vi "PROJECT_LABVIEW.vi"() -> ()   [LabVIEW 2020]
uses:
  <vilib>/Utility/NIReport.llb/Report Type.ctl
  <vilib>/DAQmx/write.llb/DAQmx Write (Analog Wfm 1Chan NSamp).vi
  <vilib>/DAQmx/read.llb/DAQmx Read (Analog 1D Wfm NChan NSamp).vi
  <vilib>/DAQmx/create/channels.llb/DAQmx Create Channel (AO-Voltage-Basic).vi
  <vilib>/DAQmx/configure/timing.llb/DAQmx Timing (Sample Clock).vi
  <vilib>/DAQmx/create/channels.llb/DAQmx Create Channel (AI-Voltage-Basic).vi
  <vilib>/DAQmx/miscellaneous.llb/DAQmx Fill In Error Info.vi
  <vilib>/measure/mascope.llb/Amplitude and Levels 1 chan.vi
  <vilib>/measure/madcrms.llb/Basic Averaged DC-RMS for 1 Chan.vi
  <vilib>/Utility/NIReport.llb/Append Report Text (str wrap).vi
  <vilib>/measure/maspectr.llb/FFT Spectrum (Mag-Phase) for 1 Chan.vi
  <vilib>/Utility/NIReport.llb/NI_report.lvclass
  <vilib>/measure/NI_MABase.lvlib
  <vilib>/measure/NI_MAPro.lvlib
  <resource>/objmgr/daqmx.rc
  <vilib>/Utility/NIReport.llb/NI_ReportGenerationCore.lvlib
panel:
  in  "error in 9":errorcluster caption="error in"
  in  "error in 8":errorcluster caption="error in"
  in  "error in 7":errorcluster caption="error in"
  in  "Tab Control":T1(tab)
  in  "number of samples 6":i32=1000
  in  "rate 6":dbl=1000.0 format="%0.2f"
  out "Generated signal (input) 6":waveform(dbl)(graph)
  in  "amplitude 6":dbl=1.0 format="%0.2p"
  in  "frequency 6":dbl=10.0 format="%0.2p"
  out "VL ARRAY 6":dbl[](array[numeric])
  in  "ADD MEASURMENT 6":bool
  out "IL 6":dbl[](array[numeric])
  in  "Current RL":dbl
  out "VS 6":dbl[](graph)
  out "VL 6":dbl[](graph)
  in  "stop 6":bool
  in  "(6) student ID 2":string
  in  "(6) student name  2":string
  in  "(6) additional comment":string
  out "Date and time 11":string
  in  "(6) student name  1":string
  in  "(6) student ID  1":string
  out "Date and time 10":string
  in  "(5) additional comment":string
  in  "(5) student ID  1":string
  in  "(5) student name  1":string
  in  "(5) student name  2":string
  in  "(5) student ID 2":string
  out "VL 5 VS IL 5":cluster{dbl[], dbl[]}(graph)
  in  "number of samples 5":i32=1000
  in  "rate 5":dbl=1000.0 format="%0.2f"
  in  "amplitude 5":dbl=1.0 format="%0.2p"
  in  "frequency 5":dbl=10.0 format="%0.2p"
  in  "ADD MEASURMENT":bool
  out "IL 5":dbl[](array[numeric])
  in  "Current RL":dbl
  out "VL 5":dbl[](array[numeric])
  out "VS-VL":dbl[](array[numeric])
  in  "CREATE REPORT 5":bool
  out "VL 5":waveform(dbl)(graph)
  out "Output (time) 3":waveform(dbl)(graph)
  out "Input(time) 3":waveform(dbl)(graph)
  out "Common gain 3":dbl[](graph)
  in  "number of samples 3":i32=1000
  in  "rate 6":dbl=1000.0
  out "frequency of sine 3":i32
  in  "amplitude 6":dbl=1.0 format="%0.2p"
  in  "From[hz] 3":i32
  in  "No of points 3":i32
  in  "To[hz] 3":i32
  in  "(3) student ID 2":string
  in  "(3) student name  2":string
  in  "(3) student name  1":string
  in  "(3) student ID  1":string
  in  "(3) additional comment  2":string
  out "Date and time 9":string
  in  "number of samples 2":i32=1000
  in  "rate 2":dbl=1000.0
  out "frequency of sine 2":i32
  in  "From[hz] 2":i32
  in  "No of points 2":i32
  in  "amplitude 2":dbl=1.0 format="%0.2p"
  in  "To[hz] 2":i32
  out "Diffrential gain 2":dbl[](graph)
  out "Output (time) 2":waveform(dbl)(graph)
  out "Input(time) 2":waveform(dbl)(graph)
  in  "(2) student ID 2":string
  in  "(2) student name 2":string
  in  "(2) student name  1":string
  in  "(2) student ID 1":string
  in  "(2) additional comment":string
  out "Date and time 8":string
  # "Report generator"
  # "Max current"
  # "Function generator"
  # "Report generator"
  # "Function generator"
  # "Output Resistance"
  # "Common mode gain"
  # "Connect output zero to Output \nConnect output to Input"
  # "Function generator"
  # "The generated signal in sweep is output1"
  # "Frequency sweep"
  # "Report generator"
  # "Differential amplification and bandwidth measurment"
  # "Connect output zero to Output \nConnect output one to Input\nThe generated signal in sweep is output1"
  # "Function generator"
  # "Frequency sweep"
  # "Report generator"
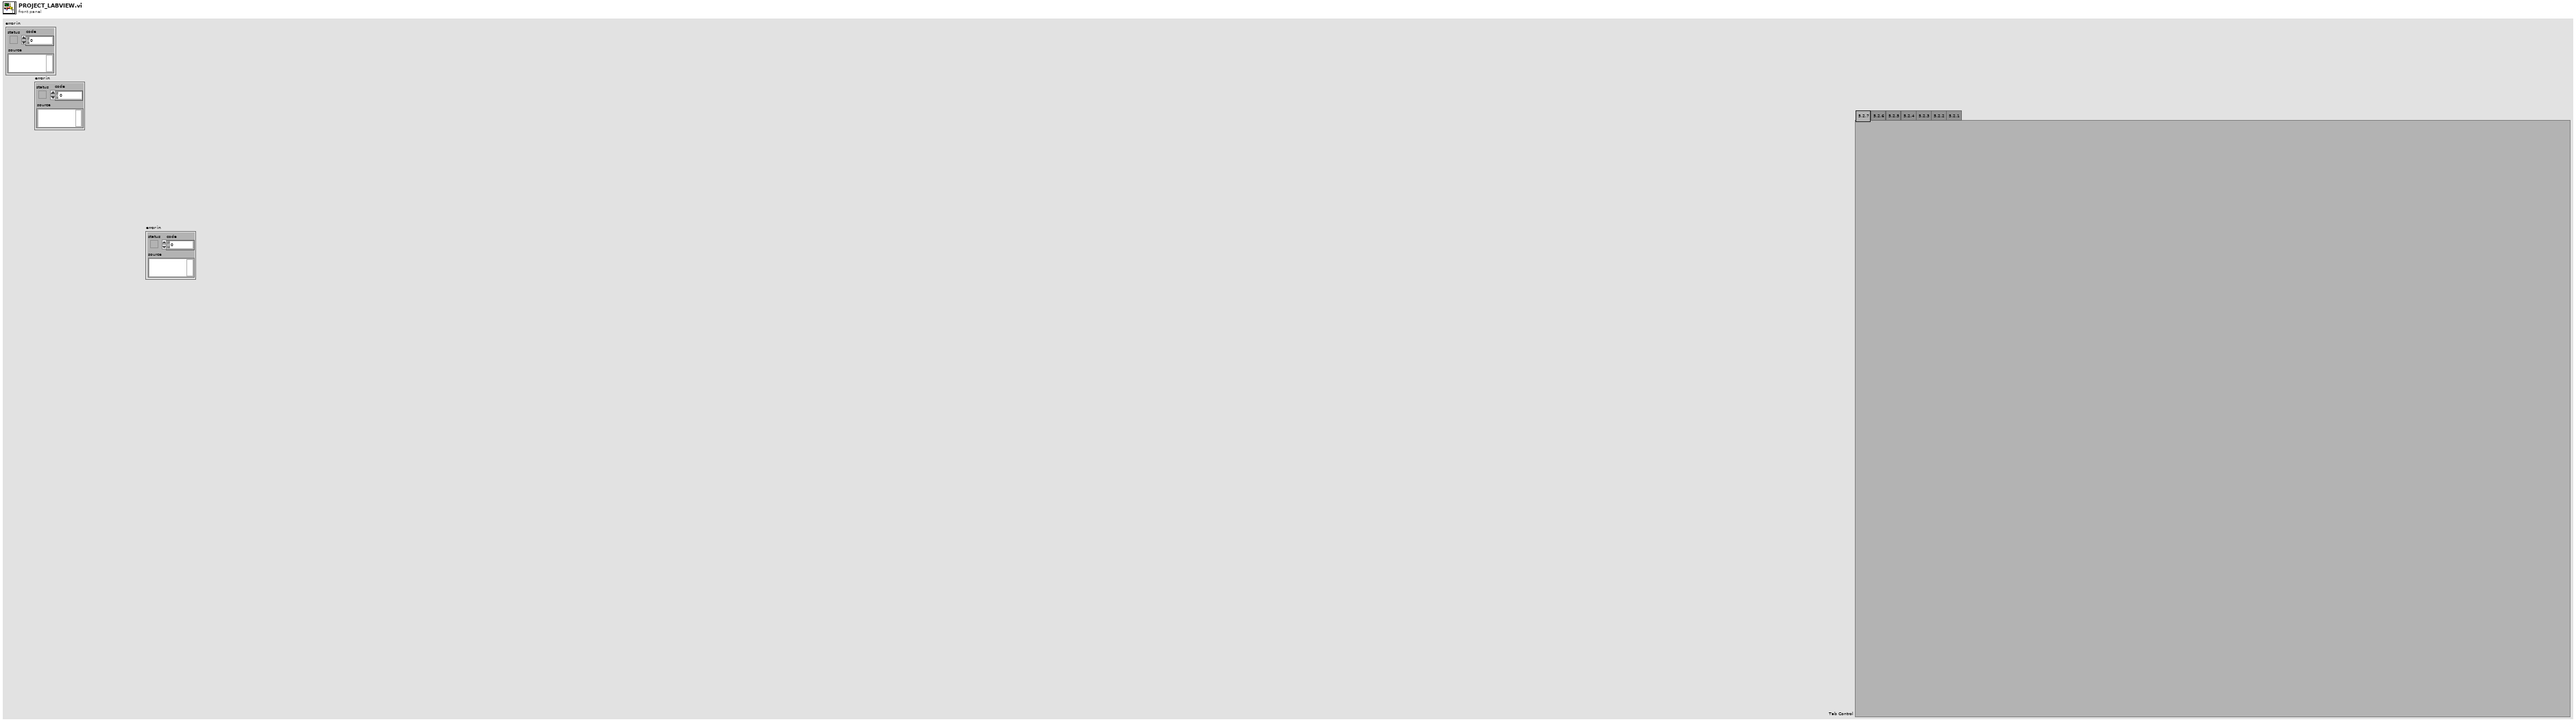
[diagram p1: front panel]
types:
  T1 = enum32{"5.2.7", "5.2.6", "5.2.5", "5.2.4", "5.2.3", "5.2.2", "5.2.1"}
  T2 = typedef "NI_ReportGenerationCore.lvlib/Report Type.ctl" = enum16{"HTML", "Word", "Excel"}
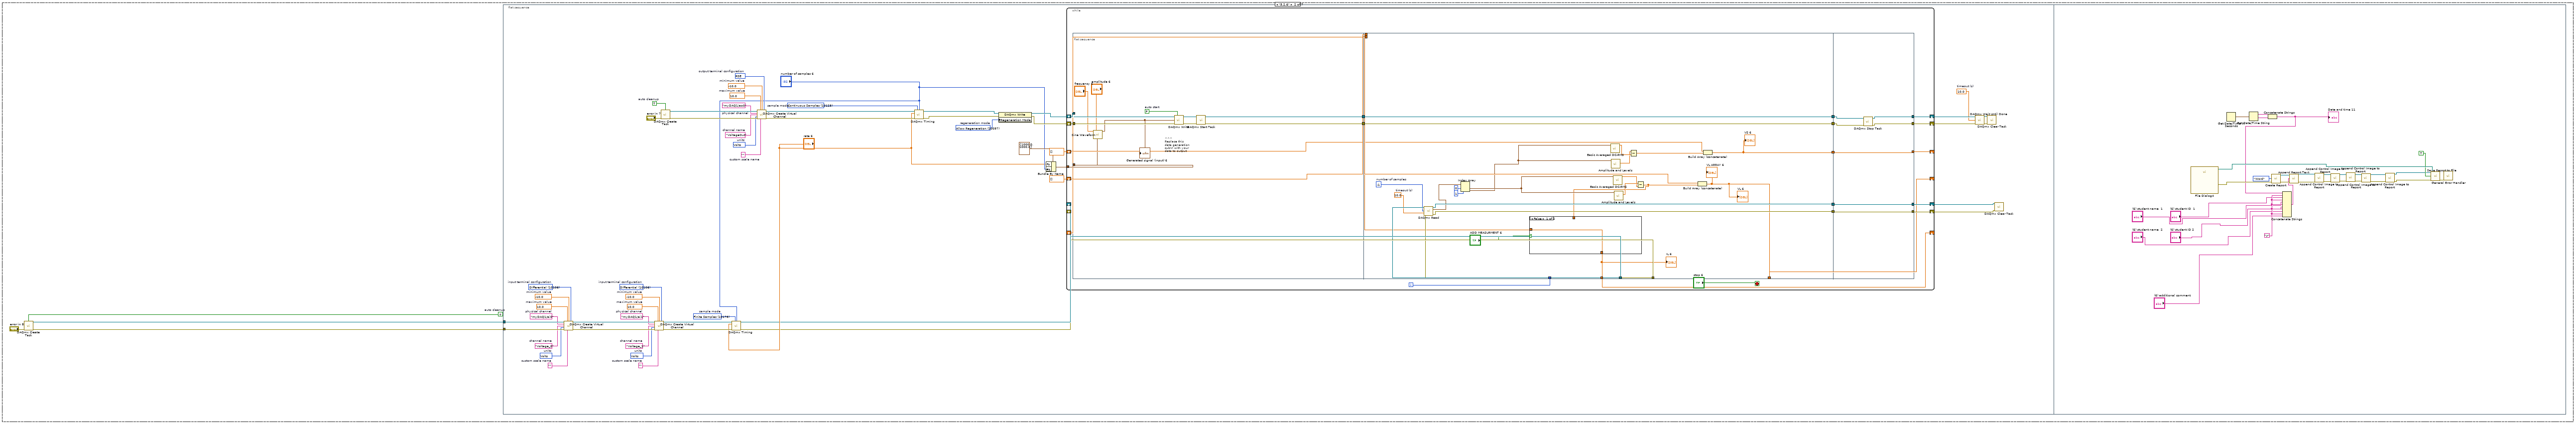
[diagram p3: hidden frame]
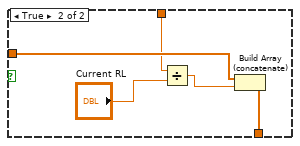
[diagram p4: hidden frame]
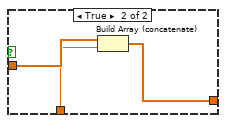
[diagram p6: hidden frame]
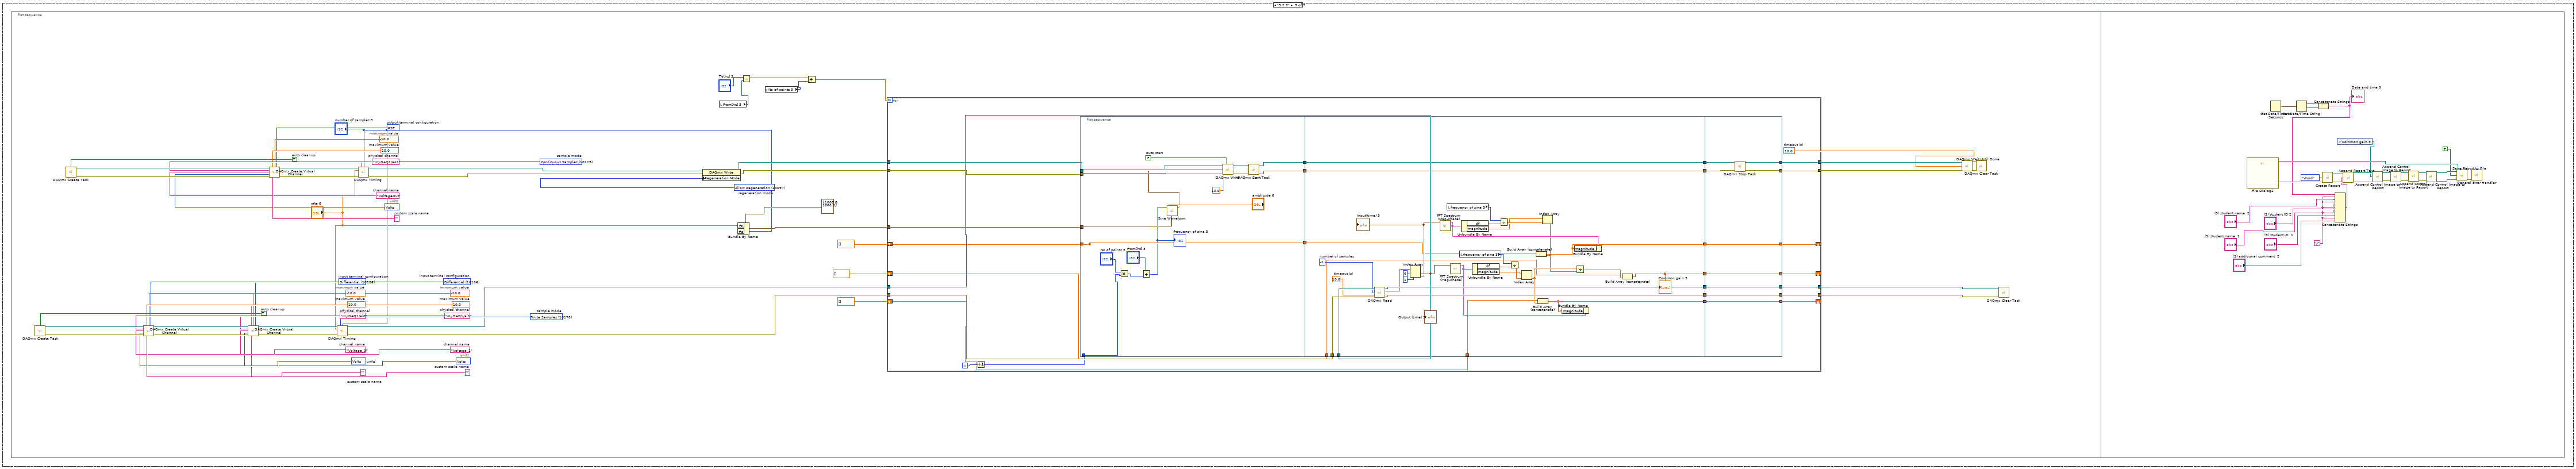
[diagram p9: hidden frame]
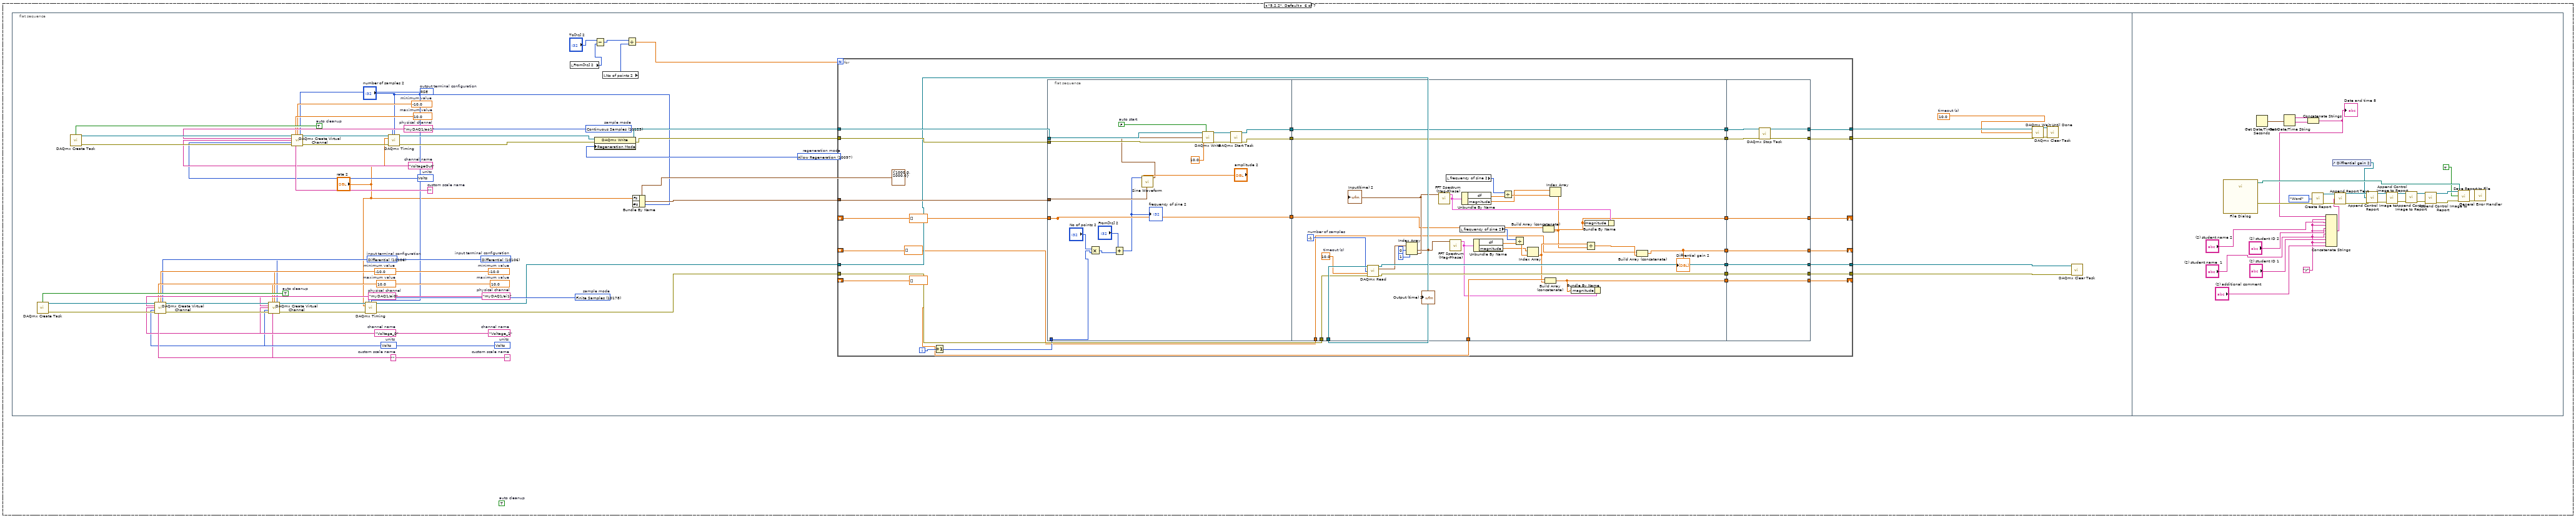
[diagram p10: hidden frame]
diagram:
  n1 = case shown="\"5.2.5\"" "Tab Control" {
    frame "5.2.7" {
    }
    frame "5.2.6" {
      w3 = TRUE  # auto cleanup
      n2 = call <vilib>:"DAQmx Create Task.vi"("auto cleanup"=w3, "error in"="error in 8") -> ("task out"=w2:refnum<k21>, "error out"=w4:errorcluster)  [unwired: 12 in]
      n3 = flat-sequence {
        tunnel: w4 -> [w35]
        tunnel: w2 -> [w34]
        frame #0 {
          w6 = 10.0  # timeout (s)
          w15 = 10178 items=["Finite Samples"=10178, "Continuous Samples"=10123, "Hardware Timed Single Point"=12522]  # sample mode
          w17 = 10106 items=["default"=-1, "RSE"=10083, "NRSE"=10078, "Differential"=10106, "Pseudodifferential"=12529]  # input terminal configuration
          w18 = 10348 items=["Volts"=10348, "From Custom Scale"=10065]  # units
          w19 = "Voltage_1"  # channel name
          w21 = ""  # custom scale name
          w22 = -10.0  # minimum value
          w23 = 10.0  # maximum value
          w24 = "myDAQ1/ai1"  # physical channel
          w26 = 10106 items=["default"=-1, "RSE"=10083, "NRSE"=10078, "Differential"=10106, "Pseudodifferential"=12529]  # input terminal configuration
          w27 = 10348 items=["Volts"=10348, "From Custom Scale"=10065]  # units
          w28 = "Voltage_0"  # channel name
          w30 = ""  # custom scale name
          w31 = -10.0  # minimum value
          w32 = 10.0  # maximum value
          w33 = "myDAQ1/ai0"  # physical channel
          w44 = 10097 items=["Allow Regeneration"=10097, "Do Not Allow Regeneration"=10158]  # regeneration mode
          w46 = 10123 items=["Finite Samples"=10178, "Continuous Samples"=10123, "Hardware Timed Single Point"=12522]  # sample mode
          w49 = 10083 items=["Default"=-1, "RSE"=10083, "Differential"=10106, "Pseudodifferential"=12529]  # output terminal configuration
          w50 = 10348 items=["Volts"=10348, "From Custom Scale"=10065]  # units
          w51 = "VoltageOut"  # channel name
          w53 = ""  # custom scale name
          w54 = -10.0  # minimum value
          w55 = 10.0  # maximum value
          w56 = "myDAQ1/ao0"  # physical channel
          w58 = TRUE  # auto cleanup
          n4 = call-poly <vilib>:"DAQmx Create Virtual Channel.vi"("task in"=w34, "maximum value"=w32, "minimum value"=w31, "input terminal configuration"=w26, "physical channels"=w33, "name to assign"=w28, "units"=w27, "error in"=w35, "custom scale name"=w30) -> ("task out"=w25:refnum<k21>, "error out"=w29:errorcluster)  [unwired: 5 in]
          n5 = call-poly <vilib>:"DAQmx Create Virtual Channel.vi"("task in"=w25, "maximum value"=w23, "minimum value"=w22, "input terminal configuration"=w17, "physical channels"=w24, "name to assign"=w19, "units"=w18, "error in"=w29, "custom scale name"=w21) -> ("task out"=w16:refnum<k21>, "error out"=w20:errorcluster)  [unwired: 5 in]
          n6 = call <vilib>:"DAQmx Create Task.vi"("auto cleanup"=w58, "error in"="error in 7") -> ("task out"=w57:refnum<k21>, "error out"=w59:errorcluster)  [unwired: 12 in]
          n7 = call-poly <vilib>:"DAQmx Timing.vi"("task/channels in"=w16, "sample mode"=w15, "samples per channel"="number of samples 6", "rate"="rate 6", "error in"=w20) -> ("task out"=w12:refnum<k21>, "error out"=w11:errorcluster)  [unwired: 9 in]
          n8 = call-poly <vilib>:"DAQmx Create Virtual Channel.vi"("task in"=w57, "maximum value"=w55, "minimum value"=w54, "output terminal configuration"=w49, "physical channels"=w56, "name to assign"=w51, "units"=w50, "error in"=w59, "custom scale name"=w53) -> ("task out"=w47:refnum<k21>, "error out"=w52:errorcluster)  [unwired: 5 in]
          n9 = call-poly <vilib>:"DAQmx Timing.vi"("task/channels in"=w47, "sample mode"=w46, "samples per channel"="number of samples 6", "rate"="rate 6", "error in"=w52) -> ("task out"=w45:refnum<k21>, "error out"=w48:errorcluster)  [unwired: 9 in]
          n10 = property class="DAQmx Write"(reference=w45, error in=w48, "Regeneration Mode"=w44) -> (reference out=w43:refnum<k21>, error out=w42:errorcluster)
          n11 = Bundle By Name(cluster=cluster{"Fs":dbl, "#s":dbl} {"Fs"=1000.0, "#s"=1000.0} ("sampling info"), "Fs"="rate 6", "#s"="number of samples 6") -> (w36:cluster{"Fs":dbl, "#s":dbl})
          n12 = while {
            tunnel: w36 -> [w74]
            shift-right: [w76] -> w39
            shift-left: w43 -> [w78]
            shift-right: [w75] -> w38
            shift-left: w42 -> [w77]
            shift-right: [w71] -> w10
            shift-left: w12 -> [w73]
            shift-right: [w70] -> w9
            shift-left: w11 -> [w72]
            shift-right: [w68] -> _
            shift-left: dbl[] [] -> [w65]
            shift-right: [w67] -> _
            shift-left: dbl[] [] -> [w66]
            shift-right: [w63] -> _
            shift-left: _ -> [w62]
            i -> [w64]
            stop <- "stop 6" stop-if-true
            n13 = flat-sequence {
              tunnel: w78 -> [w92]
              tunnel: w77 -> [w91]
              tunnel: [w90] -> w84
              tunnel: [w89] -> w83
              tunnel: w74 -> [w86]
              tunnel: w84 -> [w121]
              tunnel: [w121] -> w82
              tunnel: w83 -> [w120]
              tunnel: [w120] -> w81
              tunnel: w73 -> [w119]
              tunnel: w72 -> [w118]
              tunnel: [w115] -> w80
              tunnel: [w114] -> w79
              tunnel: [w103] -> w69
              tunnel: [w102] -> w67
              tunnel: w66 -> [w105]
              tunnel: w65 -> [w104]
              tunnel: w64 -> [_]
              tunnel: [w99] -> w63
              tunnel: w62 -> [w98]
              tunnel: [w131] -> w75
              tunnel: [w132] -> w76
              tunnel: w82 -> [w134]
              tunnel: w81 -> [w133]
              tunnel: w80 -> [w130]
              tunnel: w79 -> [w129]
              tunnel: [w130] -> w71
              tunnel: [w129] -> w70
              tunnel: w69 -> [w128]
              tunnel: [w128] -> w68
              frame #0 {
                w95 = FALSE  # auto start
                # "^^^\nReplace this\ndata generation\nsubVI with your\ndata to output"
                n14 = call <vilib>:"Sine Waveform.vi"("sampling info"=w86, "amplitude"="amplitude 6", "frequency"="frequency 6") -> ("signal out"=w85:waveform(dbl))  [unwired: 7 in, 1 out]
                "Generated signal (input) 6" <- w85
                n15 = call-poly <vilib>:"DAQmx Write.vi"("task/channels in"=w92, "auto start"=w95, "data"=w85, "error in"=w91) -> ("task out"=w94:refnum<k21>, "error out"=w93:errorcluster)  [unwired: 9 in, 1 out]
                n16 = call <vilib>:"DAQmx Start Task.vi"("task/channels in"=w94, "error in"=w93) -> ("task out"=w90:refnum<k21>, "error out"=w89:errorcluster)  [unwired: 12 in]
              }
              frame #1 {
                w116 = 10.0  # timeout (s)
                w117 = -1  # number of samples
                n17 = call-poly <vilib>:"DAQmx Read.vi"("task/channels in"=w119, "number of samples per channel"=w117, "timeout"=w116, "error in"=w118) -> ("task out"=w115:refnum<k21>, "data"=w113:waveform(dbl)[], "error out"=w114:errorcluster)  [unwired: 9 in]
                n18 = Index Array(array=w113, index #1=0 ("index"), index #2=1 ("index")) -> (element #1=w101:waveform(dbl), element #2=w100:waveform(dbl))
                n19 = call-poly <vilib>:"Basic Averaged DC-RMS.vi"("signal in"=w100) -> ("DC value"=w108:dbl)  [unwired: 7 in, 3 out]
                n20 = call-poly <vilib>:"Amplitude and Levels.vi"("signal in"=w100) -> ("high state level"=w107:dbl)  [unwired: 7 in, 3 out]
                n21 = call-poly <vilib>:"Basic Averaged DC-RMS.vi"("signal in"=w101) -> ("DC value"=w109:dbl)  [unwired: 7 in, 3 out]
                n22 = call-poly <vilib>:"Amplitude and Levels.vi"("signal in"=w101) -> ("high state level"=w110:dbl)  [unwired: 7 in, 3 out]
                n23 = Subtract(x=w107, y=w108) -> (x-y=w106:dbl)
                n24 = Subtract(x=w110, y=w109) -> (x-y=w96:dbl)
                n25 = case shown="False" "ADD MEASURMENT 6" {
                  tunnel: [w122 w127] -> w99
                  tunnel: w98 -> [w122 w126]
                  tunnel: w96 -> [_ w125]
                  frame False {
                  }
                  frame True {
                    n26 = Divide(x=w125, y="Current RL") -> (x/y=w124:dbl)
                    n27 = Build Array (concatenate)(w126, w124) -> (w127:dbl[])
                  }
                }
                "IL 6" <- w99
                n28 = Build Array (concatenate)(w105, w96) -> (w102:dbl[])
                "VL 6" <- w102
                "VL ARRAY 6" <- w102
                n29 = Build Array (concatenate)(w104, w106) -> (w103:dbl[])
                "VS 6" <- w103
              }
              frame #2 {
                n30 = call <vilib>:"DAQmx Stop Task.vi"("task/channels in"=w134, "error in"=w133) -> ("task out"=w132:refnum<k21>, "error out"=w131:errorcluster)  [unwired: 12 in]
              }
            }
          }
          n31 = call <vilib>:"DAQmx Wait Until Done.vi"("task/channels in"=w39, "timeout (sec)"=w6, "error in"=w38) -> ("task out"=w41:refnum<k21>, "error out"=w40:errorcluster)  [unwired: 11 in]
          n32 = call <vilib>:"DAQmx Clear Task.vi"("task in"=w41, "error in"=w40) -> ()  [unwired: 13 in, 1 out]
          n33 = call <vilib>:"DAQmx Clear Task.vi"("task in"=w10, "error in"=w9) -> ()  [unwired: 13 in, 1 out]
        }
        frame #1 {
          w156 = "\r"
          n34 = call "File Dialog4"() -> ("selected path"=w159:path, "error out"=w158:errorcluster)  [unwired: 12 in, 2 out]
          n35 = Get Date/Time In Seconds() -> (seconds since 1Jan1904=w164:timestamp)
          n36 = Get Date/Time String(seconds (now)=w164) -> (date string=w162:string, time string=w163:string)  [unwired: 2 in]
          n37 = Concatenate Strings(w162, w163) -> (w139:string)
          "Date and time 11" <- w139
          n38 = call <vilib>:"Create Report.vi"("report type"=Report_Type."Word", "error in (no error)"=w158) -> ("report out"=w160:refnum<class "NI_report.lvclass">, "error out"=w161:errorcluster)  [unwired: 12 in]
          n39 = Concatenate Strings(w139, w156, "(6) student ID  1", w156, "(6) student name  1", w156, "(6) student ID 2", w156, "(6) student name  2", w156, "(6) additional comment") -> (w153:string)
          n40 = call-poly <vilib>:"Append Report Text.vi"("report in"=w160, "text"=w153, "error in (no error)"=w161) -> ("report out"=w146:refnum<class "NI_report.lvclass">, "error out"=w145:errorcluster)  [unwired: 9 in, 2 out]
          n41 = call-dynamic "Append Control Image to Report.vi"("report in"=w146, "error in (no error)"=w145) -> ("report out"=w148:refnum<class "NI_report.lvclass">, "error out"=w147:errorcluster)  [unwired: 10 in, 2 out]
          n42 = call-dynamic "Append Control Image to Report.vi"("report in"=w148, "error in (no error)"=w147) -> ("report out"=w149:refnum<class "NI_report.lvclass">, "error out"=w150:errorcluster)  [unwired: 10 in, 2 out]
          n43 = call-dynamic "Append Control Image to Report.vi"("report in"=w149, "error in (no error)"=w150) -> ("report out"=w152:refnum<class "NI_report.lvclass">, "error out"=w151:errorcluster)  [unwired: 10 in, 2 out]
          n44 = call-dynamic "Append Control Image to Report.vi"("report in"=w152, "error in (no error)"=w151) -> ("report out"=w138:refnum<class "NI_report.lvclass">, "error out"=w137:errorcluster)  [unwired: 10 in, 2 out]
          n45 = call-dynamic "Append Control Image to Report.vi"("report in"=w138, "error in (no error)"=w137) -> ("report out"=w136:refnum<class "NI_report.lvclass">, "error out"=w135:errorcluster)  [unwired: 10 in, 2 out]
          n46 = call-dynamic "Save Report to File.vi"("report in"=w136, "report file path"=w159, "prompt to replace? (F)"=TRUE, "error in (no error)"=w135) -> ("error out"=w154:errorcluster)  [unwired: 10 in, 1 out]
          n47 = call <vilib>:"General Error Handler.vi"("error in (no error)"=w154) -> ()  [unwired: 10 in, 5 out]
        }
      }
    }
    frame "5.2.5" {
      w166 = 10106 items=["default"=-1, "RSE"=10083, "NRSE"=10078, "Differential"=10106, "Pseudodifferential"=12529]  # input terminal configuration
      w167 = 10348 items=["Volts"=10348, "From Custom Scale"=10065]  # units
      w168 = "Voltage_0"  # channel name
      w170 = ""  # custom scale name
      w171 = -10.0  # minimum value
      w172 = 10.0  # maximum value
      w173 = "myDAQ1/ai0"  # physical channel
      n48 = call-poly <vilib>:"DAQmx Create Virtual Channel.vi"("maximum value"=w172, "minimum value"=w171, "input terminal configuration"=w166, "physical channels"=w173, "name to assign"=w168, "units"=w167, "custom scale name"=w170) -> ("task out"=w165:refnum<k21>, "error out"=w169:errorcluster)  [unwired: 7 in]
      n49 = flat-sequence {
        tunnel: w169 -> [w191]
        tunnel: w165 -> [w190]
        frame #0 {
          w180 = 10178 items=["Finite Samples"=10178, "Continuous Samples"=10123, "Hardware Timed Single Point"=12522]  # sample mode
          w182 = 10106 items=["default"=-1, "RSE"=10083, "NRSE"=10078, "Differential"=10106, "Pseudodifferential"=12529]  # input terminal configuration
          w183 = 10348 items=["Volts"=10348, "From Custom Scale"=10065]  # units
          w184 = "Voltage_1"  # channel name
          w186 = ""  # custom scale name
          w187 = -10.0  # minimum value
          w188 = 10.0  # maximum value
          w189 = "myDAQ1/ai1"  # physical channel
          w201 = 10097 items=["Allow Regeneration"=10097, "Do Not Allow Regeneration"=10158]  # regeneration mode
          w203 = 10123 items=["Finite Samples"=10178, "Continuous Samples"=10123, "Hardware Timed Single Point"=12522]  # sample mode
          w206 = 10083 items=["Default"=-1, "RSE"=10083, "Differential"=10106, "Pseudodifferential"=12529]  # output terminal configuration
          w207 = 10348 items=["Volts"=10348, "From Custom Scale"=10065]  # units
          w208 = "VoltageOut"  # channel name
          w210 = ""  # custom scale name
          w211 = -10.0  # minimum value
          w212 = 10.0  # maximum value
          w213 = "myDAQ1/ao0"  # physical channel
          w215 = TRUE  # auto cleanup
          n50 = call-poly <vilib>:"DAQmx Create Virtual Channel.vi"("task in"=w190, "maximum value"=w188, "minimum value"=w187, "input terminal configuration"=w182, "physical channels"=w189, "name to assign"=w184, "units"=w183, "error in"=w191, "custom scale name"=w186) -> ("task out"=w181:refnum<k21>, "error out"=w185:errorcluster)  [unwired: 5 in]
          n51 = call <vilib>:"DAQmx Create Task.vi"("auto cleanup"=w215, "error in"="error in 9") -> ("task out"=w214:refnum<k21>, "error out"=w216:errorcluster)  [unwired: 12 in]
          n52 = call-poly <vilib>:"DAQmx Timing.vi"("task/channels in"=w181, "sample mode"=w180, "samples per channel"="number of samples 5", "rate"="rate 5", "error in"=w185) -> ("task out"=w177:refnum<k21>, "error out"=w176:errorcluster)  [unwired: 9 in]
          n53 = call-poly <vilib>:"DAQmx Create Virtual Channel.vi"("task in"=w214, "maximum value"=w212, "minimum value"=w211, "output terminal configuration"=w206, "physical channels"=w213, "name to assign"=w208, "units"=w207, "error in"=w216, "custom scale name"=w210) -> ("task out"=w204:refnum<k21>, "error out"=w209:errorcluster)  [unwired: 5 in]
          n54 = call-poly <vilib>:"DAQmx Timing.vi"("task/channels in"=w204, "sample mode"=w203, "samples per channel"="number of samples 5", "rate"="rate 5", "error in"=w209) -> ("task out"=w202:refnum<k21>, "error out"=w205:errorcluster)  [unwired: 9 in]
          n55 = property class="DAQmx Write"(reference=w202, error in=w205, "Regeneration Mode"=w201) -> (reference out=w200:refnum<k21>, error out=w199:errorcluster)
          n56 = Bundle By Name(cluster=cluster{"Fs":dbl, "#s":dbl} {"Fs"=1000.0, "#s"=1000.0} ("sampling info"), "Fs"="rate 5", "#s"="number of samples 5") -> (w192:cluster{"Fs":dbl, "#s":dbl})
          n57 = while {
            tunnel: [w232] -> w194
            tunnel: w192 -> [w231]
            shift-right: [w234] -> w196
            shift-left: w200 -> [w236]
            shift-right: [w233] -> w195
            shift-left: w199 -> [w235]
            shift-right: [w228] -> w175
            shift-left: w177 -> [w230]
            shift-right: [w227] -> w174
            shift-left: w176 -> [w229]
            shift-right: [w225] -> _
            shift-left: _ -> [w222]
            shift-right: [w224] -> _
            shift-left: _ -> [w223]
            shift-right: [w220] -> _
            shift-left: _ -> [w219]
            i -> [w221]
            stop <- "CREATE REPORT 5" stop-if-true
            w232 = 10.0  # timeout (s)
            n58 = flat-sequence {
              tunnel: w236 -> [w250]
              tunnel: w235 -> [w249]
              tunnel: [w248] -> w242
              tunnel: [w247] -> w241
              tunnel: w231 -> [w244]
              tunnel: w242 -> [w277]
              tunnel: [w277] -> w240
              tunnel: w241 -> [w276]
              tunnel: [w276] -> w239
              tunnel: w230 -> [w275]
              tunnel: w229 -> [w274]
              tunnel: [w271] -> w238
              tunnel: [w270] -> w237
              tunnel: [w260] -> w226
              tunnel: [w254] -> w224
              tunnel: w223 -> [w266]
              tunnel: w222 -> [w265]
              tunnel: w221 -> [_]
              tunnel: [w259] -> w220
              tunnel: w219 -> [w262]
              tunnel: [w295] -> w233
              tunnel: [w296] -> w234
              tunnel: w240 -> [w298]
              tunnel: w239 -> [w297]
              tunnel: w238 -> [w294]
              tunnel: w237 -> [w293]
              tunnel: [w294] -> w228
              tunnel: [w293] -> w227
              tunnel: w226 -> [w292]
              tunnel: [w292] -> w225
              frame #0 {
                w253 = FALSE  # auto start
                # "^^^\nReplace this\ndata generation\nsubVI with your\ndata to output"
                n59 = call <vilib>:"Sine Waveform.vi"("sampling info"=w244, "amplitude"="amplitude 5", "frequency"="frequency 5") -> ("signal out"=w243:waveform(dbl))  [unwired: 7 in, 1 out]
                n60 = call-poly <vilib>:"DAQmx Write.vi"("task/channels in"=w250, "auto start"=w253, "data"=w243, "error in"=w249) -> ("task out"=w252:refnum<k21>, "error out"=w251:errorcluster)  [unwired: 9 in, 1 out]
                n61 = call <vilib>:"DAQmx Start Task.vi"("task/channels in"=w252, "error in"=w251) -> ("task out"=w248:refnum<k21>, "error out"=w247:errorcluster)  [unwired: 12 in]
              }
              frame #1 {
                w272 = 10.0  # timeout (s)
                w273 = -1  # number of samples
                n62 = call-poly <vilib>:"DAQmx Read.vi"("task/channels in"=w275, "number of samples per channel"=w273, "timeout"=w272, "error in"=w274) -> ("task out"=w271:refnum<k21>, "data"=w269:waveform(dbl)[], "error out"=w270:errorcluster)  [unwired: 9 in]
                n63 = Index Array(array=w269, index #1=0 ("index"), index #2=1 ("index")) -> (element #1=w264:waveform(dbl), element #2=w263:waveform(dbl))
                "VL 5" <- w264
                n64 = call-poly <vilib>:"Amplitude and Levels.vi"("signal in"=w264) -> ("amplitude"=w256:dbl)  [unwired: 7 in, 3 out]
                n65 = case shown="True" "ADD MEASURMENT" {
                  tunnel: [w286 w291] -> w259
                  tunnel: w262 -> [w286 w290]
                  tunnel: w256 -> [_ w289]
                  frame False {
                  }
                  frame True {
                    n66 = Divide(x=w289, y="Current RL") -> (x/y=w288:dbl)
                    n67 = Build Array (concatenate)(w290, w288) -> (w291:dbl[])
                  }
                }
                "IL 5" <- w259
                n68 = call-poly <vilib>:"Amplitude and Levels.vi"("signal in"=w263) -> ("amplitude"=w255:dbl)  [unwired: 7 in, 3 out]
                n69 = Subtract(x=w255, y=w256) -> (x-y=w261:dbl)
                n70 = case shown="False" "ADD MEASURMENT" {
                  tunnel: w265 -> [w282 w285]
                  tunnel: w261 -> [_ w284]
                  tunnel: [w282 w283] -> w260
                  frame False {
                  }
                  frame True {
                    n71 = Build Array (concatenate)(w285, w284) -> (w283:dbl[])
                  }
                }
                "VS-VL" <- w260
                n72 = case shown="True" "ADD MEASURMENT" {
                  tunnel: w266 -> [w278 w281]
                  tunnel: [w278 w280] -> w254
                  tunnel: w256 -> [_ w279]
                  frame False {
                  }
                  frame True {
                    n73 = Build Array (concatenate)(w281, w279) -> (w280:dbl[])
                  }
                }
                "VL 5" <- w254
                n74 = Bundle(w254, w259) -> (→"VL 5 VS IL 5":cluster{dbl[], dbl[]})  [unwired: 1 in]
              }
              frame #2 {
                n75 = call <vilib>:"DAQmx Stop Task.vi"("task/channels in"=w298, "error in"=w297) -> ("task out"=w296:refnum<k21>, "error out"=w295:errorcluster)  [unwired: 12 in]
              }
            }
          }
          n76 = call <vilib>:"DAQmx Wait Until Done.vi"("task/channels in"=w196, "timeout (sec)"=w194, "error in"=w195) -> ("task out"=w198:refnum<k21>, "error out"=w197:errorcluster)  [unwired: 11 in]
          n77 = call <vilib>:"DAQmx Clear Task.vi"("task in"=w198, "error in"=w197) -> ()  [unwired: 13 in, 1 out]
          n78 = call <vilib>:"DAQmx Clear Task.vi"("task in"=w175, "error in"=w174) -> ()  [unwired: 13 in, 1 out]
        }
        frame #1 {
          w325 = "\r"
          n79 = call "File Dialog3"() -> ("selected path"=w328:path, "error out"=w327:errorcluster)  [unwired: 12 in, 2 out]
          n80 = Get Date/Time In Seconds() -> (seconds since 1Jan1904=w333:timestamp)
          n81 = Get Date/Time String(seconds (now)=w333) -> (date string=w331:string, time string=w332:string)  [unwired: 2 in]
          n82 = Concatenate Strings(w331, w332) -> (w308:string)
          "Date and time 10" <- w308
          n83 = call <vilib>:"Create Report.vi"("report type"=Report_Type."Word", "error in (no error)"=w327) -> ("report out"=w329:refnum<class "NI_report.lvclass">, "error out"=w330:errorcluster)  [unwired: 12 in]
          n84 = Concatenate Strings(w308, w325, "(5) student ID  1", w325, "(5) student name  1", w325, "(5) student ID 2", w325, "(5) student name  2", w325, "(5) additional comment") -> (w322:string)
          n85 = call-poly <vilib>:"Append Report Text.vi"("report in"=w329, "text"=w322, "error in (no error)"=w330) -> ("report out"=w315:refnum<class "NI_report.lvclass">, "error out"=w314:errorcluster)  [unwired: 9 in, 2 out]
          n86 = control-ref of="IL 5"() -> (w304:refnum<vi>)
          n87 = call-dynamic "Append Control Image to Report.vi"("report in"=w315, "ctrl reference"=w304, "error in (no error)"=w314) -> ("report out"=w317:refnum<class "NI_report.lvclass">, "error out"=w316:errorcluster)  [unwired: 9 in, 2 out]
          n88 = control-ref of="VL 5"() -> (w305:refnum<vi>)
          n89 = call-dynamic "Append Control Image to Report.vi"("report in"=w317, "ctrl reference"=w305, "error in (no error)"=w316) -> ("report out"=w318:refnum<class "NI_report.lvclass">, "error out"=w319:errorcluster)  [unwired: 9 in, 2 out]
          n90 = control-ref of="VS-VL"() -> (w306:refnum<vi>)
          n91 = call-dynamic "Append Control Image to Report.vi"("report in"=w318, "ctrl reference"=w306, "error in (no error)"=w319) -> ("report out"=w321:refnum<class "NI_report.lvclass">, "error out"=w320:errorcluster)  [unwired: 9 in, 2 out]
          n92 = control-ref of="Current RL"() -> (w307:refnum<vi>)
          n93 = call-dynamic "Append Control Image to Report.vi"("report in"=w321, "ctrl reference"=w307, "error in (no error)"=w320) -> ("report out"=w303:refnum<class "NI_report.lvclass">, "error out"=w302:errorcluster)  [unwired: 9 in, 2 out]
          n94 = control-ref of="VL 5 VS IL 5"() -> (w299:refnum<vi>)
          n95 = call-dynamic "Append Control Image to Report.vi"("report in"=w303, "ctrl reference"=w299, "error in (no error)"=w302) -> ("report out"=w301:refnum<class "NI_report.lvclass">, "error out"=w300:errorcluster)  [unwired: 9 in, 2 out]
          n96 = call-dynamic "Save Report to File.vi"("report in"=w301, "report file path"=w328, "prompt to replace? (F)"=TRUE, "error in (no error)"=w300) -> ("error out"=w323:errorcluster)  [unwired: 10 in, 1 out]
          n97 = call <vilib>:"General Error Handler.vi"("error in (no error)"=w323) -> ()  [unwired: 10 in, 5 out]
        }
      }
    }
    frame "5.2.4" {
    }
    frame "5.2.3" {
      n98 = flat-sequence {
        frame #0 {
          w342 = 10.0  # timeout (s)
          w349 = 10178 items=["Finite Samples"=10178, "Continuous Samples"=10123, "Hardware Timed Single Point"=12522]  # sample mode
          w351 = 10106 items=["default"=-1, "RSE"=10083, "NRSE"=10078, "Differential"=10106, "Pseudodifferential"=12529]  # input terminal configuration
          w352 = 10348 items=["Volts"=10348, "From Custom Scale"=10065]  # units
          w353 = "Voltage_1"  # channel name
          w355 = ""  # custom scale name
          w356 = -10.0  # minimum value
          w357 = 10.0  # maximum value
          w358 = "myDAQ1/ai1"  # physical channel
          w360 = 10106 items=["default"=-1, "RSE"=10083, "NRSE"=10078, "Differential"=10106, "Pseudodifferential"=12529]  # input terminal configuration
          w361 = 10348 items=["Volts"=10348, "From Custom Scale"=10065]  # units
          w362 = "Voltage_0"  # channel name
          w364 = ""  # custom scale name
          w365 = -10.0  # minimum value
          w366 = 10.0  # maximum value
          w367 = "myDAQ1/ai0"  # physical channel
          w369 = TRUE  # auto cleanup
          w379 = 10097 items=["Allow Regeneration"=10097, "Do Not Allow Regeneration"=10158]  # regeneration mode
          w381 = 10123 items=["Finite Samples"=10178, "Continuous Samples"=10123, "Hardware Timed Single Point"=12522]  # sample mode
          w384 = 10083 items=["Default"=-1, "RSE"=10083, "Differential"=10106, "Pseudodifferential"=12529]  # output terminal configuration
          w385 = 10348 items=["Volts"=10348, "From Custom Scale"=10065]  # units
          w386 = "VoltageOut"  # channel name
          w388 = ""  # custom scale name
          w389 = -10.0  # minimum value
          w390 = 10.0  # maximum value
          w391 = "myDAQ1/ao1"  # physical channel
          w393 = TRUE  # auto cleanup
          n99 = call <vilib>:"DAQmx Create Task.vi"("auto cleanup"=w369) -> ("task out"=w368:refnum<k21>, "error out"=w370:errorcluster)  [unwired: 13 in]
          n100 = call <vilib>:"DAQmx Create Task.vi"("auto cleanup"=w393) -> ("task out"=w392:refnum<k21>, "error out"=w394:errorcluster)  [unwired: 13 in]
          n101 = call-poly <vilib>:"DAQmx Create Virtual Channel.vi"("task in"=w368, "maximum value"=w366, "minimum value"=w365, "input terminal configuration"=w360, "physical channels"=w367, "name to assign"=w362, "units"=w361, "error in"=w370, "custom scale name"=w364) -> ("task out"=w359:refnum<k21>, "error out"=w363:errorcluster)  [unwired: 5 in]
          n102 = call-poly <vilib>:"DAQmx Create Virtual Channel.vi"("task in"=w359, "maximum value"=w357, "minimum value"=w356, "input terminal configuration"=w351, "physical channels"=w358, "name to assign"=w353, "units"=w352, "error in"=w363, "custom scale name"=w355) -> ("task out"=w350:refnum<k21>, "error out"=w354:errorcluster)  [unwired: 5 in]
          n103 = call-poly <vilib>:"DAQmx Create Virtual Channel.vi"("task in"=w392, "maximum value"=w390, "minimum value"=w389, "output terminal configuration"=w384, "physical channels"=w391, "name to assign"=w386, "units"=w385, "error in"=w394, "custom scale name"=w388) -> ("task out"=w382:refnum<k21>, "error out"=w387:errorcluster)  [unwired: 5 in]
          n104 = call-poly <vilib>:"DAQmx Timing.vi"("task/channels in"=w350, "sample mode"=w349, "samples per channel"="number of samples 3", "rate"="rate 6", "error in"=w354) -> ("task out"=w346:refnum<k21>, "error out"=w345:errorcluster)  [unwired: 9 in]
          n105 = call-poly <vilib>:"DAQmx Timing.vi"("task/channels in"=w382, "sample mode"=w381, "samples per channel"="number of samples 3", "rate"="rate 6", "error in"=w387) -> ("task out"=w380:refnum<k21>, "error out"=w383:errorcluster)  [unwired: 9 in]
          n106 = property class="DAQmx Write"(reference=w380, error in=w383, "Regeneration Mode"=w379) -> (reference out=w374:refnum<k21>, error out=w373:errorcluster)
          n107 = local read "From[hz] 3"() -> (w337:i32)
          n108 = Bundle By Name(cluster=cluster{"Fs":dbl, "#s":dbl} {"Fs"=1000.0, "#s"=1000.0} ("sampling info"), "Fs"="rate 6", "#s"="number of samples 3") -> (w371:cluster{"Fs":dbl, "#s":dbl})
          n109 = Subtract(x="To[hz] 3", y=w337) -> (x-y=w334:i32)
          n110 = local read "No of points 3"() -> (w335:i32)
          n111 = Divide(x=w334, y=w335) -> (x/y=w336:dbl)
          n112 = for {
            N: w336 -> [_]
            tunnel: w371 -> [w411]
            tunnel: w374 -> [w413]
            tunnel: [w415] -> w376
            tunnel: w373 -> [w412]
            tunnel: [w414] -> w375
            tunnel: w346 -> [w410]
            tunnel: [w408] -> w344
            tunnel: w345 -> [w409]
            tunnel: [w407] -> w343
            shift-right: [w404] -> _
            shift-left: dbl[] [] -> [w402]
            shift-right: [w400] -> _
            shift-left: dbl[] [] -> [w398]
            shift-right: [w396] -> _
            shift-left: dbl[] [] -> [w395]
            i -> [w406]
            n113 = Increment(x=w406) -> (x+1=w405:i32)
            n114 = flat-sequence {
              tunnel: [w435] -> w421
              tunnel: [w434] -> w420
              tunnel: w413 -> [w433]
              tunnel: w412 -> [w432]
              tunnel: w411 -> [w431]
              tunnel: w405 -> [w428]
              tunnel: [w423] -> _
              tunnel: [w423] -> w399
              tunnel: w398 -> [w423]
              tunnel: w421 -> [w470]
              tunnel: [w470] -> w419
              tunnel: w420 -> [w469]
              tunnel: [w469] -> w418
              tunnel: w410 -> [w468]
              tunnel: w409 -> [w465]
              tunnel: [w464] -> w417
              tunnel: [w463] -> w416
              tunnel: [w445] -> w403
              tunnel: w402 -> [w455]
              tunnel: [w446] -> w401
              tunnel: w399 -> [w450]
              tunnel: [w440] -> w397
              tunnel: w395 -> [w439]
              tunnel: [w476] -> w414
              tunnel: [w477] -> w415
              tunnel: w419 -> [w479]
              tunnel: w418 -> [w478]
              tunnel: w417 -> [w475]
              tunnel: w416 -> [w474]
              tunnel: [w475] -> w408
              tunnel: [w474] -> w407
              tunnel: [w473] -> w404
              tunnel: w403 -> [w473]
              tunnel: w401 -> [w472]
              tunnel: [w472] -> w400
              tunnel: [w471] -> w396
              tunnel: w397 -> [w471]
              frame #0 {
                w436 = FALSE  # auto start
                n115 = Multiply(x="No of points 3", y=w428) -> (x*y=w426:i32)
                n116 = Add(x="From[hz] 3", y=w426) -> (x+y=w422:i32)
                "frequency of sine 3" <- w422
                n117 = call <vilib>:"Sine Waveform.vi"("sampling info"=w431, "amplitude"="amplitude 6", "frequency"=w422) -> ("signal out"=w429:waveform(dbl))  [unwired: 7 in, 1 out]
                n118 = call-poly <vilib>:"DAQmx Write.vi"("task/channels in"=w433, "auto start"=w436, "data"=w429, "timeout"=10.0, "error in"=w432) -> ("task out"=w437:refnum<k21>, "error out"=w438:errorcluster)  [unwired: 8 in, 1 out]
                n119 = call <vilib>:"DAQmx Start Task.vi"("task/channels in"=w437, "error in"=w438) -> ("task out"=w435:refnum<k21>, "error out"=w434:errorcluster)  [unwired: 12 in]
              }
              frame #1 {
                w466 = 10.0  # timeout (s)
                w467 = -1  # number of samples
                n120 = call-poly <vilib>:"DAQmx Read.vi"("task/channels in"=w468, "number of samples per channel"=w467, "timeout"=w466, "error in"=w465) -> ("task out"=w464:refnum<k21>, "data"=w462:waveform(dbl)[], "error out"=w463:errorcluster)  [unwired: 9 in]
                n121 = Index Array(array=w462, index #1=0 ("index"), index #2=1 ("index")) -> (element #1=w459:waveform(dbl), element #2=w451:waveform(dbl))
                "Output (time) 3" <- w459
                "Input(time) 3" <- w451
                n122 = call-poly <vilib>:"FFT Spectrum (Mag-Phase).vi"("time signal"=w451) -> ("magnitude"=w447:cluster{"f0":dbl, "df":dbl, "magnitude":dbl[]})  [unwired: 6 in, 4 out]
                n123 = local read "frequency of sine 3"() -> (w449:i32)
                n124 = call-poly <vilib>:"FFT Spectrum (Mag-Phase).vi"("time signal"=w459) -> ("magnitude"=w444:cluster{"f0":dbl, "df":dbl, "magnitude":dbl[]})  [unwired: 6 in, 4 out]
                n125 = local read "frequency of sine 3"() -> (w448:i32)
                n126 = Unbundle By Name(w447) -> ("df"=w454:dbl, "magnitude"=w452:dbl[])
                n127 = Unbundle By Name(w444) -> ("df"=w458:dbl, "magnitude"=w456:dbl[])
                n128 = Divide(x=w449, y=w454) -> (x/y=w453:dbl)
                n129 = Divide(x=w448, y=w458) -> (x/y=w457:dbl)
                n130 = Index Array(array=w456, index=w457) -> (element=w443:dbl)
                n131 = Build Array (concatenate)(w455, w443) -> (w445:dbl[])
                n132 = Index Array(array=w452, index=w453) -> (element=w442:dbl)
                n133 = Build Array (concatenate)(w450, w442) -> (w446:dbl[])
                n134 = Bundle By Name(cluster=w444, "magnitude"=w445) -> ()  [unwired: 1 out]
                n135 = Bundle By Name(cluster=w447, "magnitude"=w446) -> ()  [unwired: 1 out]
                n136 = Divide(x=w443, y=w442) -> (x/y=w441:dbl)
                n137 = Build Array (concatenate)(w439, w441) -> (w440:dbl[])
                "Common gain 3" <- w440
              }
              frame #2 {
                n138 = call <vilib>:"DAQmx Stop Task.vi"("task/channels in"=w479, "error in"=w478) -> ("task out"=w477:refnum<k21>, "error out"=w476:errorcluster)  [unwired: 12 in]
              }
            }
          }
          n139 = call <vilib>:"DAQmx Wait Until Done.vi"("task/channels in"=w376, "timeout (sec)"=w342, "error in"=w375) -> ("task out"=w377:refnum<k21>, "error out"=w378:errorcluster)  [unwired: 11 in]
          n140 = call <vilib>:"DAQmx Clear Task.vi"("task in"=w377, "error in"=w378) -> ()  [unwired: 13 in, 1 out]
          n141 = call <vilib>:"DAQmx Clear Task.vi"("task in"=w344, "error in"=w343) -> ()  [unwired: 13 in, 1 out]
        }
        frame #1 {
          w493 = "\r"
          n142 = call "File Dialog2"() -> ("selected path"=w496:path, "error out"=w495:errorcluster)  [unwired: 12 in, 2 out]
          n143 = Get Date/Time In Seconds() -> (seconds since 1Jan1904=w508:timestamp)
          n144 = Get Date/Time String(seconds (now)=w508) -> (date string=w506:string, time string=w507:string)  [unwired: 2 in]
          n145 = Concatenate Strings(w506, w507) -> (w491:string)
          "Date and time 9" <- w491
          n146 = call <vilib>:"Create Report.vi"("report type"=Report_Type."Word", "error in (no error)"=w495) -> ("report out"=w497:refnum<class "NI_report.lvclass">, "error out"=w499:errorcluster)  [unwired: 12 in]
          n147 = Concatenate Strings(w491, w493, "(3) student name  2", w493, "(3) student ID 2", w493, "(3) student name  1", w493, "(3) student ID  1", w493, "(3) additional comment  2") -> (w489:string)
          n148 = control-ref of="Common gain 3"() -> (w480:refnum<vi>)
          n149 = call-poly <vilib>:"Append Report Text.vi"("report in"=w497, "text"=w489, "error in (no error)"=w499) -> ("report out"=w482:refnum<class "NI_report.lvclass">, "error out"=w481:errorcluster)  [unwired: 9 in, 2 out]
          n150 = call-dynamic "Append Control Image to Report.vi"("report in"=w482, "ctrl reference"=w480, "error in (no error)"=w481) -> ("report out"=w484:refnum<class "NI_report.lvclass">, "error out"=w483:errorcluster)  [unwired: 9 in, 2 out]
          n151 = call-dynamic "Append Control Image to Report.vi"("report in"=w484, "error in (no error)"=w483) -> ("report out"=w485:refnum<class "NI_report.lvclass">, "error out"=w486:errorcluster)  [unwired: 10 in, 2 out]
          n152 = call-dynamic "Append Control Image to Report.vi"("report in"=w485, "error in (no error)"=w486) -> ("report out"=w488:refnum<class "NI_report.lvclass">, "error out"=w487:errorcluster)  [unwired: 10 in, 2 out]
          n153 = call-dynamic "Append Control Image to Report.vi"("report in"=w488, "error in (no error)"=w487) -> ("report out"=w498:refnum<class "NI_report.lvclass">, "error out"=w500:errorcluster)  [unwired: 10 in, 2 out]
          n154 = call-dynamic "Save Report to File.vi"("report in"=w498, "report file path"=w496, "prompt to replace? (F)"=TRUE, "error in (no error)"=w500) -> ("error out"=w490:errorcluster)  [unwired: 10 in, 1 out]
          n155 = call <vilib>:"General Error Handler.vi"("error in (no error)"=w490) -> ()  [unwired: 10 in, 5 out]
        }
      }
    }
    frame "5.2.2", Default {
      (unwired) TRUE  # auto cleanup
      n156 = flat-sequence {
        frame #0 {
          w517 = 10.0  # timeout (s)
          w524 = 10178 items=["Finite Samples"=10178, "Continuous Samples"=10123, "Hardware Timed Single Point"=12522]  # sample mode
          w526 = 10106 items=["default"=-1, "RSE"=10083, "NRSE"=10078, "Differential"=10106, "Pseudodifferential"=12529]  # input terminal configuration
          w527 = 10348 items=["Volts"=10348, "From Custom Scale"=10065]  # units
          w528 = "Voltage_1"  # channel name
          w530 = ""  # custom scale name
          w531 = -10.0  # minimum value
          w532 = 10.0  # maximum value
          w533 = "myDAQ1/ai1"  # physical channel
          w535 = 10106 items=["default"=-1, "RSE"=10083, "NRSE"=10078, "Differential"=10106, "Pseudodifferential"=12529]  # input terminal configuration
          w536 = 10348 items=["Volts"=10348, "From Custom Scale"=10065]  # units
          w537 = "Voltage_0"  # channel name
          w539 = ""  # custom scale name
          w540 = -10.0  # minimum value
          w541 = 10.0  # maximum value
          w542 = "myDAQ1/ai0"  # physical channel
          w544 = TRUE  # auto cleanup
          w554 = 10097 items=["Allow Regeneration"=10097, "Do Not Allow Regeneration"=10158]  # regeneration mode
          w556 = 10123 items=["Finite Samples"=10178, "Continuous Samples"=10123, "Hardware Timed Single Point"=12522]  # sample mode
          w559 = 10083 items=["Default"=-1, "RSE"=10083, "Differential"=10106, "Pseudodifferential"=12529]  # output terminal configuration
          w560 = 10348 items=["Volts"=10348, "From Custom Scale"=10065]  # units
          w561 = "VoltageOut"  # channel name
          w563 = ""  # custom scale name
          w564 = -10.0  # minimum value
          w565 = 10.0  # maximum value
          w566 = "myDAQ1/ao1"  # physical channel
          w568 = TRUE  # auto cleanup
          n157 = call <vilib>:"DAQmx Create Task.vi"("auto cleanup"=w544) -> ("task out"=w543:refnum<k21>, "error out"=w545:errorcluster)  [unwired: 13 in]
          n158 = call <vilib>:"DAQmx Create Task.vi"("auto cleanup"=w568) -> ("task out"=w567:refnum<k21>, "error out"=w569:errorcluster)  [unwired: 13 in]
          n159 = call-poly <vilib>:"DAQmx Create Virtual Channel.vi"("task in"=w543, "maximum value"=w541, "minimum value"=w540, "input terminal configuration"=w535, "physical channels"=w542, "name to assign"=w537, "units"=w536, "error in"=w545, "custom scale name"=w539) -> ("task out"=w534:refnum<k21>, "error out"=w538:errorcluster)  [unwired: 5 in]
          n160 = call-poly <vilib>:"DAQmx Create Virtual Channel.vi"("task in"=w534, "maximum value"=w532, "minimum value"=w531, "input terminal configuration"=w526, "physical channels"=w533, "name to assign"=w528, "units"=w527, "error in"=w538, "custom scale name"=w530) -> ("task out"=w525:refnum<k21>, "error out"=w529:errorcluster)  [unwired: 5 in]
          n161 = call-poly <vilib>:"DAQmx Create Virtual Channel.vi"("task in"=w567, "maximum value"=w565, "minimum value"=w564, "output terminal configuration"=w559, "physical channels"=w566, "name to assign"=w561, "units"=w560, "error in"=w569, "custom scale name"=w563) -> ("task out"=w557:refnum<k21>, "error out"=w562:errorcluster)  [unwired: 5 in]
          n162 = call-poly <vilib>:"DAQmx Timing.vi"("task/channels in"=w525, "sample mode"=w524, "samples per channel"="number of samples 2", "rate"="rate 2", "error in"=w529) -> ("task out"=w521:refnum<k21>, "error out"=w520:errorcluster)  [unwired: 9 in]
          n163 = call-poly <vilib>:"DAQmx Timing.vi"("task/channels in"=w557, "sample mode"=w556, "samples per channel"="number of samples 2", "rate"="rate 2", "error in"=w562) -> ("task out"=w555:refnum<k21>, "error out"=w558:errorcluster)  [unwired: 9 in]
          n164 = local read "From[hz] 2"() -> (w511:i32)
          n165 = property class="DAQmx Write"(reference=w555, error in=w558, "Regeneration Mode"=w554) -> (reference out=w549:refnum<k21>, error out=w548:errorcluster)
          n166 = Subtract(x="To[hz] 2", y=w511) -> (x-y=w509:i32)
          n167 = local read "No of points 2"() -> (w510:i32)
          n168 = Divide(x=w509, y=w510) -> (x/y=w516:dbl)
          n169 = Bundle By Name(cluster=cluster{"Fs":dbl, "#s":dbl} {"Fs"=1000.0, "#s"=1000.0} ("sampling info"), "Fs"="rate 2", "#s"="number of samples 2") -> (w546:cluster{"Fs":dbl, "#s":dbl})
          n170 = for {
            N: w516 -> [_]
            tunnel: w546 -> [w586]
            tunnel: w549 -> [w588]
            tunnel: [w590] -> w551
            tunnel: w548 -> [w587]
            tunnel: [w589] -> w550
            tunnel: w521 -> [w585]
            tunnel: [w583] -> w519
            tunnel: w520 -> [w584]
            tunnel: [w582] -> w518
            shift-right: [w579] -> _
            shift-left: dbl[] [] -> [w577]
            shift-right: [w575] -> _
            shift-left: dbl[] [] -> [w573]
            shift-right: [w571] -> _
            shift-left: dbl[] [] -> [w570]
            i -> [w581]
            n171 = Increment(x=w581) -> (x+1=w580:i32)
            n172 = flat-sequence {
              tunnel: [w610] -> w596
              tunnel: [w609] -> w595
              tunnel: w588 -> [w608]
              tunnel: w587 -> [w607]
              tunnel: w586 -> [w606]
              tunnel: w580 -> [w603]
              tunnel: [w598] -> _
              tunnel: [w598] -> w574
              tunnel: w573 -> [w598]
              tunnel: w596 -> [w645]
              tunnel: [w645] -> w594
              tunnel: w595 -> [w644]
              tunnel: [w644] -> w593
              tunnel: w585 -> [w643]
              tunnel: w584 -> [w640]
              tunnel: [w639] -> w592
              tunnel: [w638] -> w591
              tunnel: [w620] -> w578
              tunnel: w577 -> [w630]
              tunnel: [w621] -> w576
              tunnel: w574 -> [w625]
              tunnel: [w615] -> w572
              tunnel: w570 -> [w614]
              tunnel: [w651] -> w589
              tunnel: [w652] -> w590
              tunnel: w594 -> [w654]
              tunnel: w593 -> [w653]
              tunnel: w592 -> [w650]
              tunnel: w591 -> [w649]
              tunnel: [w650] -> w583
              tunnel: [w649] -> w582
              tunnel: [w648] -> w579
              tunnel: w578 -> [w648]
              tunnel: w576 -> [w647]
              tunnel: [w647] -> w575
              tunnel: [w646] -> w571
              tunnel: w572 -> [w646]
              frame #0 {
                w611 = FALSE  # auto start
                n173 = Multiply(x="No of points 2", y=w603) -> (x*y=w601:i32)
                n174 = Add(x="From[hz] 2", y=w601) -> (x+y=w597:i32)
                "frequency of sine 2" <- w597
                n175 = call <vilib>:"Sine Waveform.vi"("sampling info"=w606, "amplitude"="amplitude 2", "frequency"=w597) -> ("signal out"=w604:waveform(dbl))  [unwired: 7 in, 1 out]
                n176 = call-poly <vilib>:"DAQmx Write.vi"("task/channels in"=w608, "auto start"=w611, "data"=w604, "timeout"=10.0, "error in"=w607) -> ("task out"=w612:refnum<k21>, "error out"=w613:errorcluster)  [unwired: 8 in, 1 out]
                n177 = call <vilib>:"DAQmx Start Task.vi"("task/channels in"=w612, "error in"=w613) -> ("task out"=w610:refnum<k21>, "error out"=w609:errorcluster)  [unwired: 12 in]
              }
              frame #1 {
                w641 = 10.0  # timeout (s)
                w642 = -1  # number of samples
                n178 = call-poly <vilib>:"DAQmx Read.vi"("task/channels in"=w643, "number of samples per channel"=w642, "timeout"=w641, "error in"=w640) -> ("task out"=w639:refnum<k21>, "data"=w637:waveform(dbl)[], "error out"=w638:errorcluster)  [unwired: 9 in]
                n179 = Index Array(array=w637, index #1=0 ("index"), index #2=1 ("index")) -> (element #1=w634:waveform(dbl), element #2=w626:waveform(dbl))
                "Output (time) 2" <- w634
                "Input(time) 2" <- w626
                n180 = call-poly <vilib>:"FFT Spectrum (Mag-Phase).vi"("time signal"=w626) -> ("magnitude"=w622:cluster{"f0":dbl, "df":dbl, "magnitude":dbl[]})  [unwired: 6 in, 4 out]
                n181 = local read "frequency of sine 2"() -> (w624:i32)
                n182 = call-poly <vilib>:"FFT Spectrum (Mag-Phase).vi"("time signal"=w634) -> ("magnitude"=w619:cluster{"f0":dbl, "df":dbl, "magnitude":dbl[]})  [unwired: 6 in, 4 out]
                n183 = local read "frequency of sine 2"() -> (w623:i32)
                n184 = Unbundle By Name(w622) -> ("df"=w629:dbl, "magnitude"=w627:dbl[])
                n185 = Unbundle By Name(w619) -> ("df"=w633:dbl, "magnitude"=w631:dbl[])
                n186 = Divide(x=w624, y=w629) -> (x/y=w628:dbl)
                n187 = Divide(x=w623, y=w633) -> (x/y=w632:dbl)
                n188 = Index Array(array=w631, index=w632) -> (element=w618:dbl)
                n189 = Build Array (concatenate)(w630, w618) -> (w620:dbl[])
                n190 = Index Array(array=w627, index=w628) -> (element=w617:dbl)
                n191 = Build Array (concatenate)(w625, w617) -> (w621:dbl[])
                n192 = Bundle By Name(cluster=w619, "magnitude"=w620) -> ()  [unwired: 1 out]
                n193 = Bundle By Name(cluster=w622, "magnitude"=w621) -> ()  [unwired: 1 out]
                n194 = Divide(x=w618, y=w617) -> (x/y=w616:dbl)
                n195 = Build Array (concatenate)(w614, w616) -> (w615:dbl[])
                "Diffrential gain 2" <- w615
              }
              frame #2 {
                n196 = call <vilib>:"DAQmx Stop Task.vi"("task/channels in"=w654, "error in"=w653) -> ("task out"=w652:refnum<k21>, "error out"=w651:errorcluster)  [unwired: 12 in]
              }
            }
          }
          n197 = call <vilib>:"DAQmx Wait Until Done.vi"("task/channels in"=w551, "timeout (sec)"=w517, "error in"=w550) -> ("task out"=w552:refnum<k21>, "error out"=w553:errorcluster)  [unwired: 11 in]
          n198 = call <vilib>:"DAQmx Clear Task.vi"("task in"=w552, "error in"=w553) -> ()  [unwired: 13 in, 1 out]
          n199 = call <vilib>:"DAQmx Clear Task.vi"("task in"=w519, "error in"=w518) -> ()  [unwired: 13 in, 1 out]
        }
        frame #1 {
          w668 = "\r"
          n200 = call "File Dialog"() -> ("selected path"=w671:path, "error out"=w670:errorcluster)  [unwired: 12 in, 2 out]
          n201 = Get Date/Time In Seconds() -> (seconds since 1Jan1904=w683:timestamp)
          n202 = Get Date/Time String(seconds (now)=w683) -> (date string=w681:string, time string=w682:string)  [unwired: 2 in]
          n203 = Concatenate Strings(w681, w682) -> (w666:string)
          "Date and time 8" <- w666
          n204 = call <vilib>:"Create Report.vi"("report type"=Report_Type."Word", "error in (no error)"=w670) -> ("report out"=w672:refnum<class "NI_report.lvclass">, "error out"=w674:errorcluster)  [unwired: 12 in]
          n205 = Concatenate Strings(w666, w668, "(2) student name 2", w668, "(2) student ID 2", w668, "(2) student name  1", w668, "(2) student ID 1", w668, "(2) additional comment") -> (w664:string)
          n206 = control-ref of="Diffrential gain 2"() -> (w655:refnum<vi>)
          n207 = call-poly <vilib>:"Append Report Text.vi"("report in"=w672, "text"=w664, "error in (no error)"=w674) -> ("report out"=w657:refnum<class "NI_report.lvclass">, "error out"=w656:errorcluster)  [unwired: 9 in, 2 out]
          n208 = call-dynamic "Append Control Image to Report.vi"("report in"=w657, "ctrl reference"=w655, "error in (no error)"=w656) -> ("report out"=w659:refnum<class "NI_report.lvclass">, "error out"=w658:errorcluster)  [unwired: 9 in, 2 out]
          n209 = call-dynamic "Append Control Image to Report.vi"("report in"=w659, "error in (no error)"=w658) -> ("report out"=w660:refnum<class "NI_report.lvclass">, "error out"=w661:errorcluster)  [unwired: 10 in, 2 out]
          n210 = call-dynamic "Append Control Image to Report.vi"("report in"=w660, "error in (no error)"=w661) -> ("report out"=w663:refnum<class "NI_report.lvclass">, "error out"=w662:errorcluster)  [unwired: 10 in, 2 out]
          n211 = call-dynamic "Append Control Image to Report.vi"("report in"=w663, "error in (no error)"=w662) -> ("report out"=w673:refnum<class "NI_report.lvclass">, "error out"=w675:errorcluster)  [unwired: 10 in, 2 out]
          n212 = call-dynamic "Save Report to File.vi"("report in"=w673, "report file path"=w671, "prompt to replace? (F)"=TRUE, "error in (no error)"=w675) -> ("error out"=w665:errorcluster)  [unwired: 10 in, 1 out]
          n213 = call <vilib>:"General Error Handler.vi"("error in (no error)"=w665) -> ()  [unwired: 10 in, 5 out]
        }
      }
    }
    frame "5.2.1" {
    }
  }
